vi "DB_EscribeTablaEquipos.vi"(8 "error in":errorcluster, 11 "Equipos":string[][](array[string])) -> (0 "error out":errorcluster, 3 "IPs":string[](array[string]))   [LabVIEW 2018]
uses:
  <vilib>/addons/database/Connection.llb/DB Tools Open Connec (Path).vi
  <vilib>/addons/database/Connection.llb/Conn Execute.vi
  <vilib>/addons/database/Recordset.llb/Rec Destroy - Connection.vi
  <vilib>/addons/database/NI_Database_API.lvlib
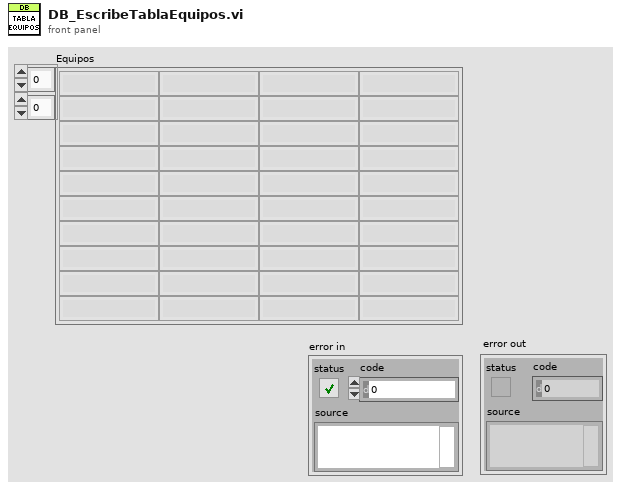
[diagram p1: front panel]
types:
  T1 = typedef "NI_Database_API.lvlib/Conn ObjectReference.ctl" = refnum<k1>
  T2 = typedef "NI_Database_API.lvlib/Rec ObjectReference.ctl" = refnum<k1>
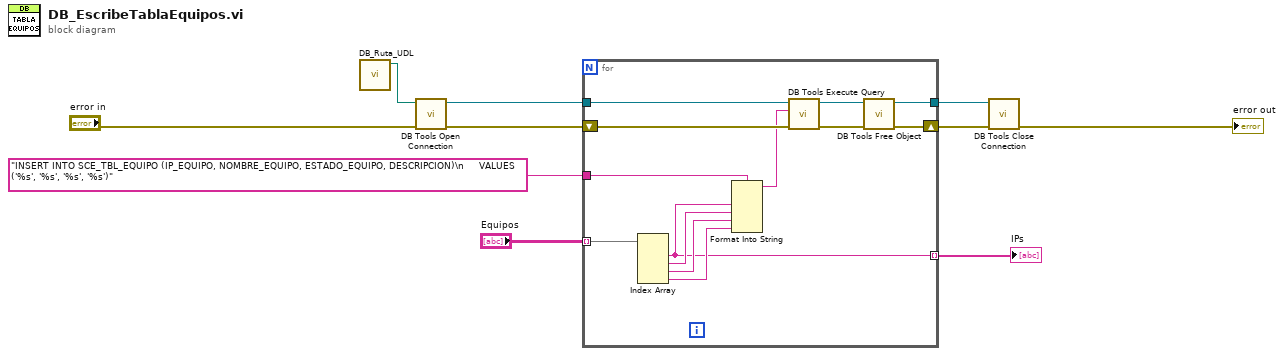
[diagram p0: block diagram]
diagram:
  n1 = call "DB_Ruta_UDL.vi"() -> ("UDL ruta"=w2:path)  [unwired: 11 in]
  n2 = call-poly <vilib>:"DB Tools Open Connection.vi"("error in (no error)"="error in", "connection information"=w2) -> ("error out"=w8:errorcluster, "connection reference"=w6:T1)  [unwired: 6 in]
  n3 = for {
    tunnel: w6 -> [w21]
    shift-right: [w22] -> w7
    shift-left: w8 -> [w23]
    tunnel: "INSERT INTO SCE_TBL_EQUIPO (IP_EQUIPO, NOMBRE_EQUIPO, ESTADO_EQUIPO, DESCRIPCION)\n     VALUES ('%s', '%s', '%s', '%s')" ("SQL") -> [w18]
    tunnel: "Equipos" -> [w16] mode=indexing
    tunnel: [w12] -> w4 mode=indexing
    tunnel: [w11] -> w1
    n4 = Index Array(array=w16) -> (element #1=w12:string, element #2=w15:string, element #3=w14:string, element #4=w13:string)  [unwired: 4 in]
    n5 = Format Into String(format string=w18, w12, w15, w14, w13) -> (resulting string=w17:string)  [unwired: 2 in, 1 out]
    n6 = call-poly <vilib>:"DB Tools Execute Query.vi"("error in (no error)"=w23, "SQL query"=w17, "connection reference"=w21) -> ("error out"=w20:errorcluster, "recordset reference"=w19:T2)  [unwired: 5 in]
    n7 = call-poly <vilib>:"DB Tools Free Object.vi"("error in (no error)"=w20, "recordset reference"=w19) -> ("error out"=w22:errorcluster, "connection reference"=w11:T1)  [unwired: 8 in]
  }
  "IPs" <- w4
  n8 = call <vilib>:"DB Tools Close Connection.vi"("error in (no error)"=w7, "connection reference"=w1) -> ("error out"=→"error out":errorcluster)  [unwired: 5 in]
